vi "Send notification.vi"(8 "error in (no error)":errorcluster, 11 "Unregister JSON in":refnum<class "Unregister JSON.lvclass">) -> (0 "error out":errorcluster, 3 "Unregister JSON out":refnum<class "Unregister JSON.lvclass">)   [LabVIEW 2020, in "wamplv.lvlib" / "Unregister JSON.lvclass"]
uses:
  Unregister JSON.lvclass
  Unregister JSON.lvclass/Unregister JSON.ctl
  Message loop classes/ErrorOrSuccess/ErrorOrSuccess.lvclass
  Message loop classes/ErrorOrSuccess JSON/ErrorOrSuccess JSON.lvclass
  C:/local/wamplv/Private/Message loop classes/ErrorOrSuccess/ErrorOrSuccess.lvclass
  C:/local/wamplv/Private/Message loop classes/ErrorOrSuccess JSON/ErrorOrSuccess JSON.lvclass
panel:
  in  "notification":refnum<class "ErrorOrSuccess JSON.lvclass">
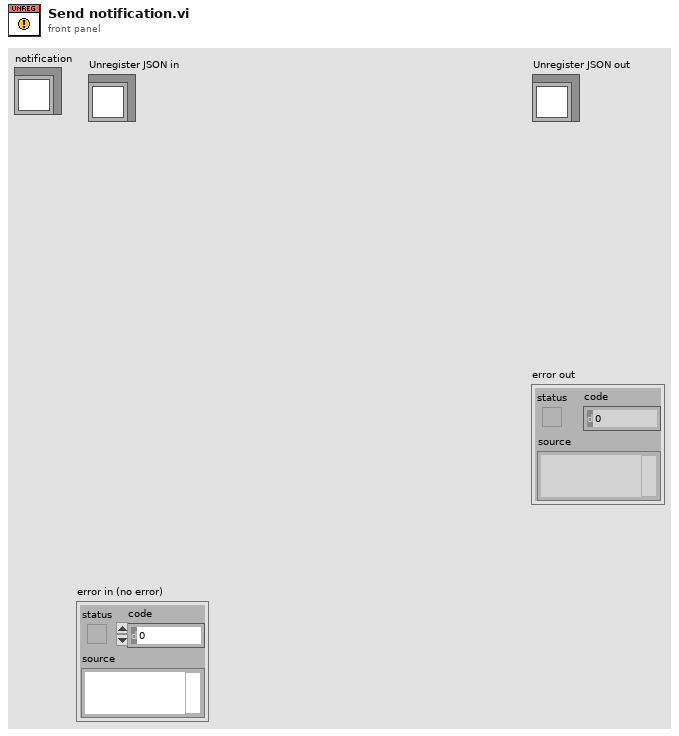
[diagram p1: front panel]
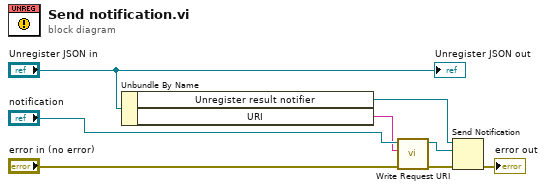
[diagram p0: block diagram]
diagram:
  n1 = Unbundle By Name("Unregister JSON in") -> ("Unregister result notifier"=w4:refnum<notifier>, "URI"=w3:string)
  n2 = call "Write Request URI.vi"("error in (no error)"="error in (no error)", "Request URI"=w3, "ErrorOrSuccess in"="notification") -> ("error out"=w1:errorcluster, "ErrorOrSuccess out"=w2:refnum<class "ErrorOrSuccess JSON.lvclass">)  [unwired: 7 in]
  n3 = Send Notification(notification=w2, notifier=w4, error in (no error)=w1) -> (error out=→"error out":errorcluster)  [unwired: 1 out]
  "Unregister JSON out" <- "Unregister JSON in"
